vi "Init.vi"(8 "error in":errorcluster, 11 "Data":variant) -> (0 "error out":errorcluster)   [LabVIEW 2010, in "Config Database.lvlib"]
doc: "This VI enqueues the named action."
uses:
  Config Database.lvlib
  Private Controls/Module Action.ctl
  Private Controls/Module Data Cluster.ctl
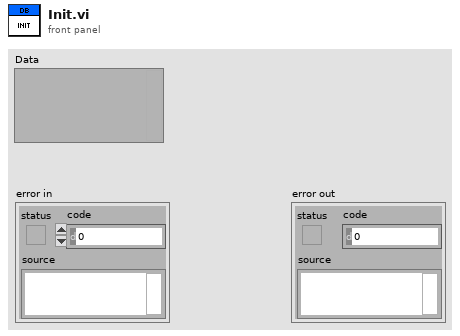
[diagram p1: front panel]
types:
  T1 = typedef "Config Database.lvlib/Module Data Cluster.ctl" = cluster{"Data":variant, "Action":T2}
  T2 = typedef "Config Database.lvlib/Module Action.ctl" = enum16{"Get balance", "Find Account", "Update balance", "Error", "Exit", "Init"}
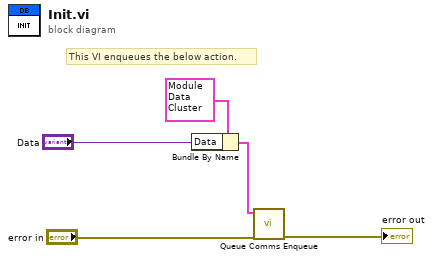
[diagram p0: block diagram]
diagram:
  # "This VI enqueues the below action."
  n1 = Bundle By Name(cluster=T1 {"Data"=variant, "Action"=enum."Init"} ("element"), "Data"="Data") -> (w1:T1)
  n2 = call "Queue Comms Enqueue.vi"("error in"="error in", "element"=w1) -> ("error out"=→"error out":errorcluster)  [unwired: 9 in]
